vi "Active Noise Control (Simulated).vi"() -> ()   [LabVIEW 2023]
doc: "This example demonstrates how to apply a filtered-x LMS adaptive filter to active noise control applications. This example simulates the primary noise with a multi-tone signal, simulates the propagation from the primary noise to the location of interest with a delay, simulates the digital-to-analog converter (DAC) and the control speaker with an FIR filter, and simulates the superposition of the noise in space at the location of interest with the addition operation.\n\nRun the VI, and the <b>Noise</b> graph in the <b>Active Noise Control</b> page displays the noise waveform at the location of interest before and after active noise control. If you change the settings for the simulated primary noise, you might need to adjust the adaptive filter parameters so that the adaptive filter converges."
uses:
  <vilib>/ptbypt/NI_PtbyPt.lvlib
  <vilib>/addons/Adaptive Filters/NI_AdaptiveFilter.lvlib
  <vilib>/Analysis/NI_AALBase.lvlib
panel:
  in  "Tab Control":enum32{"Background", "Active Noise Control"}(tab)
  in  "Primary Noise":T1(array[cluster])=[{"frequency"=120.0, "amplitude"=1.0, "phase"=55.0}, {"frequency"=240.0, "amplitude"=0.4, "phase"=134.0}, {"frequency"=360.0, "amplitude"=0.2, "phase"=110.0}]
  out "Noise":dbl[][](graph)
  in  "Step Size":dbl=0.0002 min=0.0 step=0.0001
  in  "Filter Length":i32=300 min=2
  # "Refer to the Active Noise Control topic in the LabVIEW Help for more information about the background of active noise control. Select Help>>Show Context Help and move the cursor over the VI icon of this example for more information."
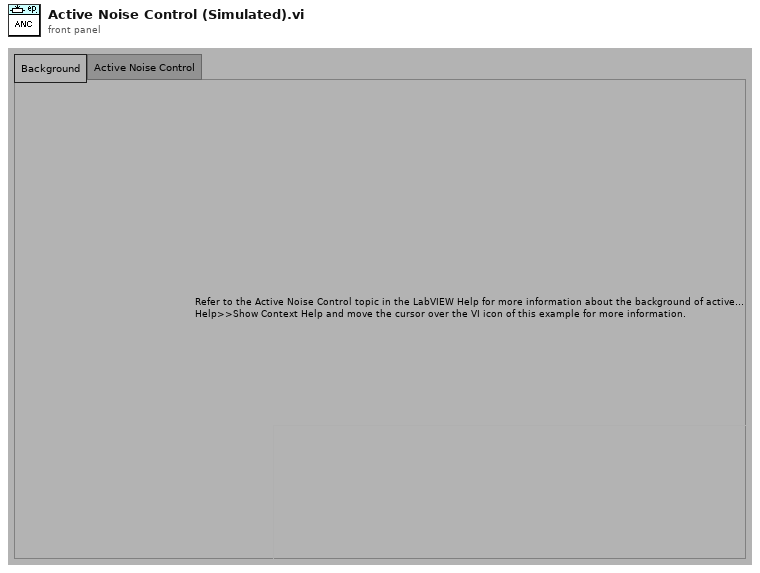
[diagram p1: front panel]
types:
  T1 = cluster{"frequency":dbl, "amplitude":dbl, "phase":dbl}[]
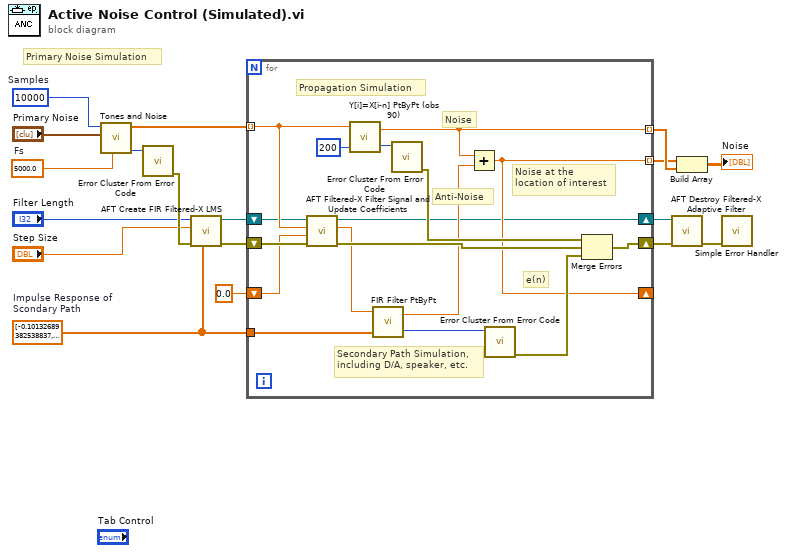
[diagram p0: block diagram]
diagram:
  w4 = 5000.0  # Fs
  w5 = 10000  # Samples
  w9 = dbl[] [-0.10132689382538837, 0.021979664110432052, 0.04315961316267942, 0.010003234659880811, -0.02453838315972942, -0.029502391384022945, -0.01133403262477631, 0.0034751099930438204, 0.0006094985078576808, -0.011755479836677067, -0.01829337481074023, -0.014559112148119285, -0.00785873219123632, -0.006510188276304974, -0.0112073117350225, -0.017047677712816157, -0.01931329338908274, -0.017522974648444132, -0.01428063109429734, -0.013219572704088585, -0.016207493968072185, -0.022197964957867387, -0.025164751702279345, -0.019917848802463393, -0.010003505438597383, -0.009047112558727675, -0.024502074398267223, -0.04349173301200617, -0.037907672601446694, 0.0005267348932624179, 0.036185298785165985, 0.01294930549478134, -0.07170984775857815, -0.12989866712754808, -0.046243113438134274, 0.1872315514487185, 0.41830304293636617, 0.45467311155623347, 0.2633211894587754, 0.010595653143360029, -0.11994589325572357, -0.09220264292519749, -0.00599216332217202, 0.035633577082091895, 0.015661295308099395, -0.01832802112927939, -0.025735352081092618, -0.008471809884706962, 0.008229490377812898, 0.009524842986507527, 0.001327605245002951, -0.0033771056761639387, 4.464155492825047e-05, 0.006565708408768082, 0.009962874867120263, 0.008639074344455794, 0.0047791927154769865, 0.001573831490921712, 0.001451693602515742, 0.004559921753410905, 0.007887958425535937, 0.007535799875060259, 0.002884203798574461, -0.001344314217800628, 0.0003799233173196481, 0.006770849192730407, 0.008993493616569854, 0.0016727113712982828, -0.0075415788358042584, -0.005082257913402113, 0.009631454746260345, 0.019115298279073174, 0.00975192801362449, -0.006673775899013366, -0.00727738852199998, 0.008282224932711251, 0.0179374280711509, 0.010111721153453304, -0.002837161239050076, -0.005248237495930041, 0.002404488060745071, 0.00887089570481903, 0.007901788010002303, 0.0027392334378310342, -0.0011633868582299584, -0.002088968488861745, -0.0012220546674807486, 0.00036348091969339437, 0.0021901096740054734, 0.0030039949540063425, 0.0012408136005707096, -0.0020922540604038317, -0.00230573461244562, 0.003782641047101538, 0.011413893200078655, 0.00989233225781435, -0.004979323980230643, -0.020788137822369376, -0.011625563465474066, 0.04926146181842194]  # Impulse Response of Scondary Path
  # "Primary Noise Simulation"
  n1 = call <vilib>:"Tones and Noise.vi"("Fs"=w4, "tones"="Primary Noise", "samples"=w5) -> ("error"=w1:i32, "tones and noise"=w3:dbl[])  [unwired: 4 in, 3 out]
  n2 = call <vilib>:"Error Cluster From Error Code.vi"("error code (0)"=w1) -> ("error out"=w18:errorcluster)  [unwired: 2 in, 6 out]
  n3 = call <vilib>:"AFT Create FIR Filtered-X LMS.vi"("secondary path"=w9, "error in (no error)"=w18, "step size"="Step Size", "filter length"="Filter Length") -> ("error out"=w11:errorcluster, "filtered-x adaptive filter out"=w14:refnum<k20>)  [unwired: 6 out]
  n4 = for {
    tunnel: w9 -> [w30]
    tunnel: w3 -> [w28] mode=indexing
    shift-right: [w29] -> _
    shift-left: 0.0 -> [w27]
    tunnel: [w29] -> w10 mode=indexing
    tunnel: [w24] -> w13 mode=indexing
    shift-right: [w26] -> w7
    shift-left: w14 -> [w22]
    shift-right: [w19] -> w8
    shift-left: w11 -> [w35]
    # "Noise at the \nlocation of interest"
    # "Anti-Noise"
    # "Noise"
    # "Propagation Simulation"
    # "e(n)"
    # "Secondary Path Simulation,\nincluding D/A, speaker, etc."
    n5 = call <vilib>:"AFT Filtered-X Filter Signal and Update Coefficients.vi"("error in (no error)"=w35, "e(n)"=w27, "x(n)"=w28, "filtered-x adaptive filter in"=w22) -> ("error out"=w33:errorcluster, "y(n)"=w25:dbl, "filtered-x adaptive filter out"=w26:refnum<k20>)  [unwired: 2 in, 3 out]
    n6 = call <vilib>:"Y[i]=X[i-n] PtByPt (obs 90).vi"("shifts: n"=200, "x"=w28) -> ("error"=w21:i32, "shifted x"=w24:dbl)  [unwired: 2 in]
    n7 = call <vilib>:"FIR Filter PtByPt.vi"("Forward Coefficients"=w30, "x"=w25) -> ("error"=w20:i32, "Filtered x"=w31:dbl)  [unwired: 1 in, 1 out]
    n8 = call <vilib>:"Error Cluster From Error Code.vi"("error code (0)"=w21) -> ("error out"=w34:errorcluster)  [unwired: 2 in, 6 out]
    n9 = Add(x=w24, y=w31) -> (x+y=w29:dbl)
    n10 = call <vilib>:"Error Cluster From Error Code.vi"("error code (0)"=w20) -> ("error out"=w32:errorcluster)  [unwired: 2 in, 6 out]
    n11 = Merge Errors(w34, w33, w32) -> (w19:errorcluster)
  }
  n12 = call <vilib>:"AFT Destroy Filtered-X Adaptive Filter.vi"("error in (no error)"=w8, "filtered-x adaptive filter in"=w7) -> ("error out"=w2:errorcluster)  [unwired: 9 out]
  n13 = Build Array(w10, w13) -> (→"Noise":dbl[][])
  n14 = call <vilib>:"Simple Error Handler.vi"("error in (no error)"=w2) -> ()  [unwired: 1 in, 8 out]
